vi "运维调试_采配水SNV2.vi"() -> ()   [LabVIEW 2016, in "PLC.lvlib"]
uses:
  PLC.lvlib
  control/switch.ctl
  <vilib>/Plasmionique/MB Master/MB_Master/MB_Master.lvclass
  <vilib>/Utility/miscctls.llb/LVPointTypeDef.ctl
  <vilib>/Plasmionique/MB Master/MB_Master_Serial/MB_Master_Serial.lvclass
  C:/Program Files (x86)/National Instruments/LabVIEW 2016/vi.lib/Plasmionique/MB Master/MB_Master/MB_Master.lvclass
  <vilib>/Plasmionique/MB Master/MB Master.lvlib
panel:
  in  "更新程序 2":T1
  out "X6":bool caption="断电检测"
  out "R13":i16
  in  "进样阀":bool
  in  "更新程序":bool
  in  "R116":i16(ring) caption="储水水体选择" items=["自来水", "采水泵"]
  out "当前启动泵号":u16(ring) items=["1号水样泵", "2号水样泵"]
  out "R113":i16 caption="储水时间设定"
  out "R25":i16
  in  "V14NC":bool
  out "R24":i16
  in  "V14NO":bool
  out "采配水版本号":string
  out "R23":i16 caption="清洗频次计数"
  out "R112":i16 caption="清洗频次设定"
  out "R22":i16
  in  "V13NC":bool
  out "R111":i16 caption="排液时间"
  out "通讯故障":bool
  out "R21":i16
  in  "V13NO":bool
  out "R20":i16
  in  "M1-2":bool
  in  "潜水泵工作模式":u16(ring) items=["泵1单泵单管路", "泵2单泵单管路", "潜水泵双泵双管路", "自吸泵双泵双管路"]
  out "X1":bool caption="进样检测"
  out "X0":bool caption="采样池液位开关"
  out "R109":i16 caption="配水时间"
  out "集成报警信息":string
  out "R108":i16 caption="自来水报警"
  out "R107":i16 caption="采水池液位报警设置"
  out "R106":i16 caption="进样超时设置"
  out "R105":i16 caption="二级清洗时间"
  out "R104":i16 caption="一级清洗时间"
  out "R103":i16 caption="外部管路清洗时间"
  out "R102":i16 caption="静置沉淀时间"
  out "R101":i16 caption="内部管路润洗时间"
  out "R100":i16 caption="外部管路润洗时间"
  out "R2":i16
  out "R1":i16
  out "多列列表框":i32(listbox)
  out "R19":i16
  in  "V6":bool
  out "R18":i16
  in  "V5":bool
  out "R17":i16
  in  "V4":bool
  out "R16":i16
  in  "V3":bool
  out "R15":i16
  in  "V2":bool
  out "R14":i16
  in  "M2":bool
  out "R12":i16
  in  "M1-1":bool
  in  "返回":bool
  in  "参数设置":bool
  in  "单步启动":bool
  in  "启动":bool
  in  "停止":bool
  # "S"
  # "次"
  # "次"
  # "S"
  # "S"
  # "S"
  # "S"
  # "S"
  # "S"
  # "S"
  # "S"
  # "S"
  # "S"
  # "S"
  # "单步计时："
  # "s"
  # "流程计时："
  # "s"
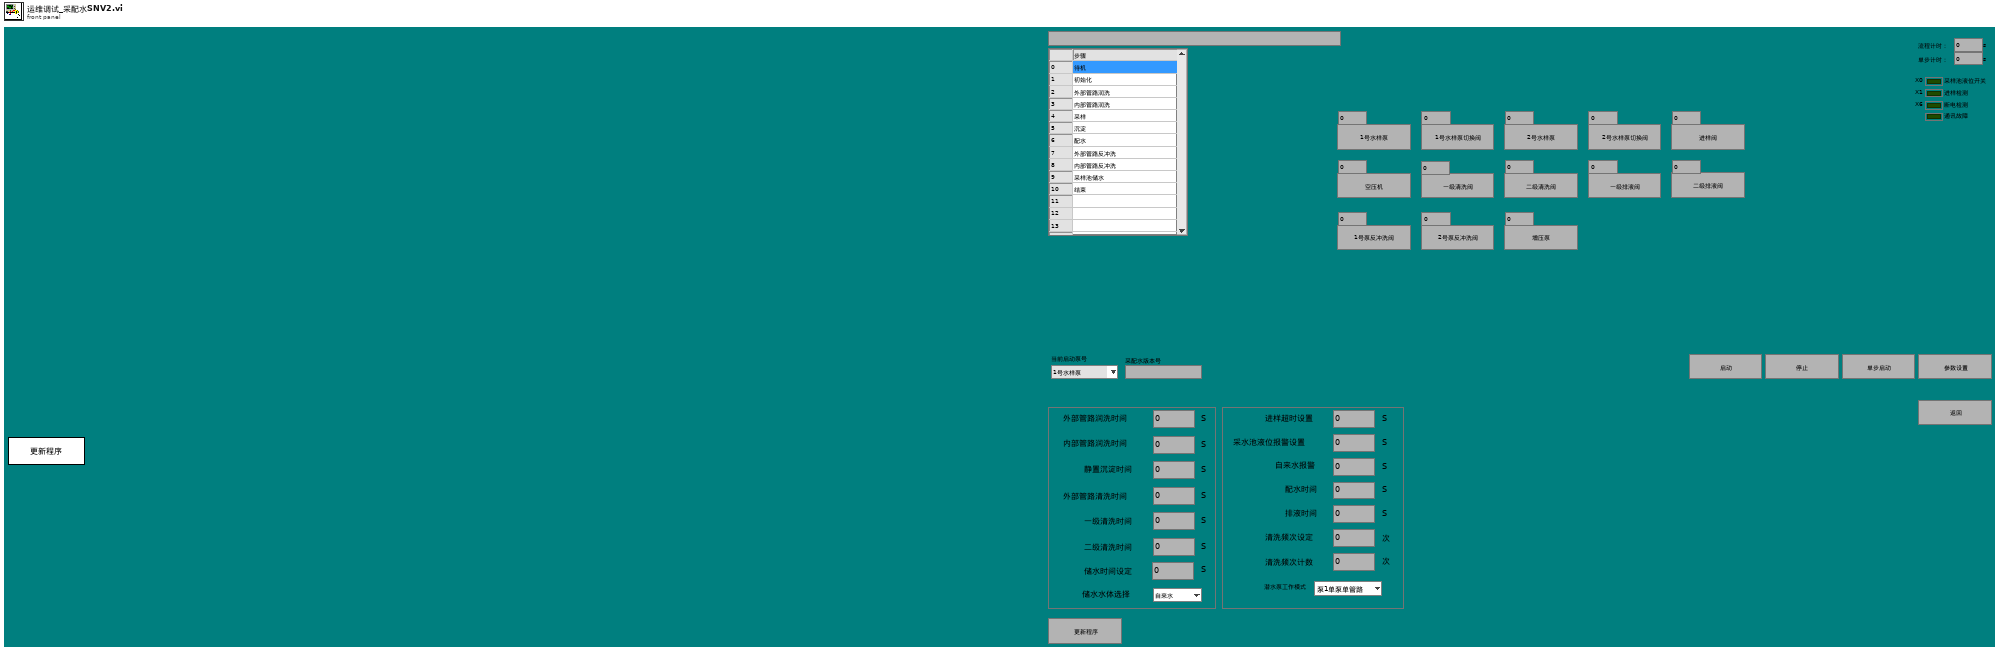
[diagram p1: front panel]
types:
  T1 = typedef "PLC.lvlib/switch.ctl" = bool
  T2 = typedef "参数.ctl" = cluster{"测试模式":enum16{"水样测试", "平行样测试", "集成干预测试", "加标回收"}, "参数启用":T3}
  T3 = typedef "启动参数.ctl" = cluster{"氨氮":bool, "总磷":bool, "总氮":bool, "多参数":bool, "CODmn":bool, "CODCr":bool, "氟化物":bool, "超标留样启用":bool}
  T4 = typedef "LVPointTypeDef.ctl" = cluster{"Horizontal":i16, "Vertical":i16}
  T5 = cluster{"R0":i16, "R1":i16, "R2":i16, "R3":i16, "R4":i16, "R5":i16, "R6":i16, "R7":i16, "R8":i16, "R9":i16, "R10":i16, "R11":i16, "R12":i16, "R13":i16, "R14":i16, "R15":i16, "R16":i16, "R17":i16, "R18":i16, "R19":i16, "R20":i16, "R21":i16, "R22":i16, "R23":i16, "R24":i16, "R25":i16, "R26":i16, "R27":i16, "R28":i16, "R29":i16, "R30":i16, "R31":i16, "R32":i16, "R33":i16, "R34":i16, "R35":i16, "R36":i16, "R37":i16, "R38":i16, "R39":i16, "R40":i16, "R41":i16, "R42":i16, "R43":i16, "R44":i16, "R45":i16, "R46":i16, "R47":i16, "R48":i16, "R49":i16, "R50":i16, "R51":i16, "R52":i16, "R53":i16, "R54":i16, "R55":i16, "R56":i16, "R57":i16, "R58":i16, "R59":i16, "R60":i16, "R61":i16, "R62":i16, "R63":i16, "R64":i16, "R65":i16, "R66":i16, "R67":i16, "R68":i16, "R69":i16, "R70":i16, "R71":i16, "R72":i16, "R73":i16, "R74":i16, "R75":i16, "R76":i16, "R77":i16, "R78":i16, "R79":i16}
  T6 = cluster{"seconds since 1Jan1904":timestamp, "table输入":string, string, "table输入":string}
  T7 = cluster{"命令":string, cluster{"starting address":u16, "holding register value":u16}}
  T8 = cluster{"命令":string, "数据":cluster{"starting address":u16, "holding register value":u16}}
  T9 = cluster{"命令":string, "数据":cluster{"starting address":u16, "holding register values":u16[]}}
  T10 = cluster{"命令":string, "data":cluster{"starting address":u16, "coil values":bool[]}}
  T11 = cluster{"测试模式":enum16{"水样测试", "平行样测试", "集成干预测试", "加标回收"}, "参数启用":T3}
  T12 = cluster{"baud rate (bps)":u32, "stop bits":u16, "parity":u16, "flow control":u16, "timeout":u32, "retries":i32}
  T13 = cluster{"starting address":u16, "holding register values":u16[]}
  T14 = cluster{"starting address":u16, "holding register value":u16}
  T15 = cluster{"starting address":u16, "coil values":bool[]}
  T16 = cluster{"Registers[0]":u16, "Registers[1]":u16, "Registers[2]":u16, "Registers[3]":u16, "Registers[4]":u16, "Registers[5]":u16, "Registers[6]":u16, "Registers[7]":u16, "Registers[8]":u16, "Registers[9]":u16, "Registers[10]":u16, "Registers[11]":u16, "Registers[12]":u16, "Registers[13]":u16, "Registers[14]":u16, "Registers[15]":u16, "Registers[16]":u16, "Registers[17]":u16, "Registers[18]":u16, "Registers[19]":u16, "Registers[20]":u16, "Registers[21]":u16, "Registers[22]":u16, "Registers[23]":u16, "Registers[24]":u16, "Registers[25]":u16, "Registers[26]":u16, "Registers[27]":u16, "Registers[28]":u16, "Registers[29]":u16, "Registers[30]":u16, "Registers[31]":u16, "Registers[32]":u16, "Registers[33]":u16, "Registers[34]":u16, "Registers[35]":u16, "Registers[36]":u16, "Registers[37]":u16, "Registers[38]":u16, "Registers[39]":u16, "Registers[40]":u16, "Registers[41]":u16, "Registers[42]":u16, "Registers[43]":u16, "Registers[44]":u16, "Registers[45]":u16, "Registers[46]":u16, "Registers[47]":u16, "Registers[48]":u16, "Registers[49]":u16, "Registers[50]":u16, "Registers[51]":u16, "Registers[52]":u16, "Registers[53]":u16, "Registers[54]":u16, "Registers[55]":u16, "Registers[56]":u16, "Registers[57]":u16, "Registers[58]":u16, "Registers[59]":u16, "Registers[60]":u16, "Registers[61]":u16, "Registers[62]":u16, "Registers[63]":u16, "Registers[64]":u16, "Registers[65]":u16, "Registers[66]":u16, "Registers[67]":u16, "Registers[68]":u16, "Registers[69]":u16, "Registers[70]":u16, "Registers[71]":u16, "Registers[72]":u16, "Registers[73]":u16, "Registers[74]":u16, "Registers[75]":u16, "Registers[76]":u16, "Registers[77]":u16, "Registers[78]":u16, "Registers[79]":u16}
  T17 = cluster{"Registers[0]":u16, "Registers[1]":u16, "Registers[2]":u16, "Registers[3]":u16, "Registers[4]":u16, "Registers[5]":u16}
  T18 = cluster{"Registers[0]":u16, "Registers[1]":u16, "Registers[2]":u16, "Registers[3]":u16, "Registers[4]":u16, "Registers[5]":u16, "Registers[6]":u16, "Registers[7]":u16, "Registers[8]":u16, "Registers[9]":u16, "Registers[10]":u16, "Registers[11]":u16, "Registers[12]":u16, "Registers[13]":u16, "Registers[14]":u16, "Registers[15]":u16, "Registers[16]":u16, "Registers[17]":u16, "Registers[18]":u16, "Registers[19]":u16, "Registers[20]":u16, "Registers[21]":u16, "Registers[22]":u16, "Registers[23]":u16, "Registers[24]":u16, "Registers[25]":u16, "Registers[26]":u16, "Registers[27]":u16, "Registers[28]":u16, "Registers[29]":u16, "Registers[30]":u16, "Registers[31]":u16, "Registers[32]":u16, "Registers[33]":u16}
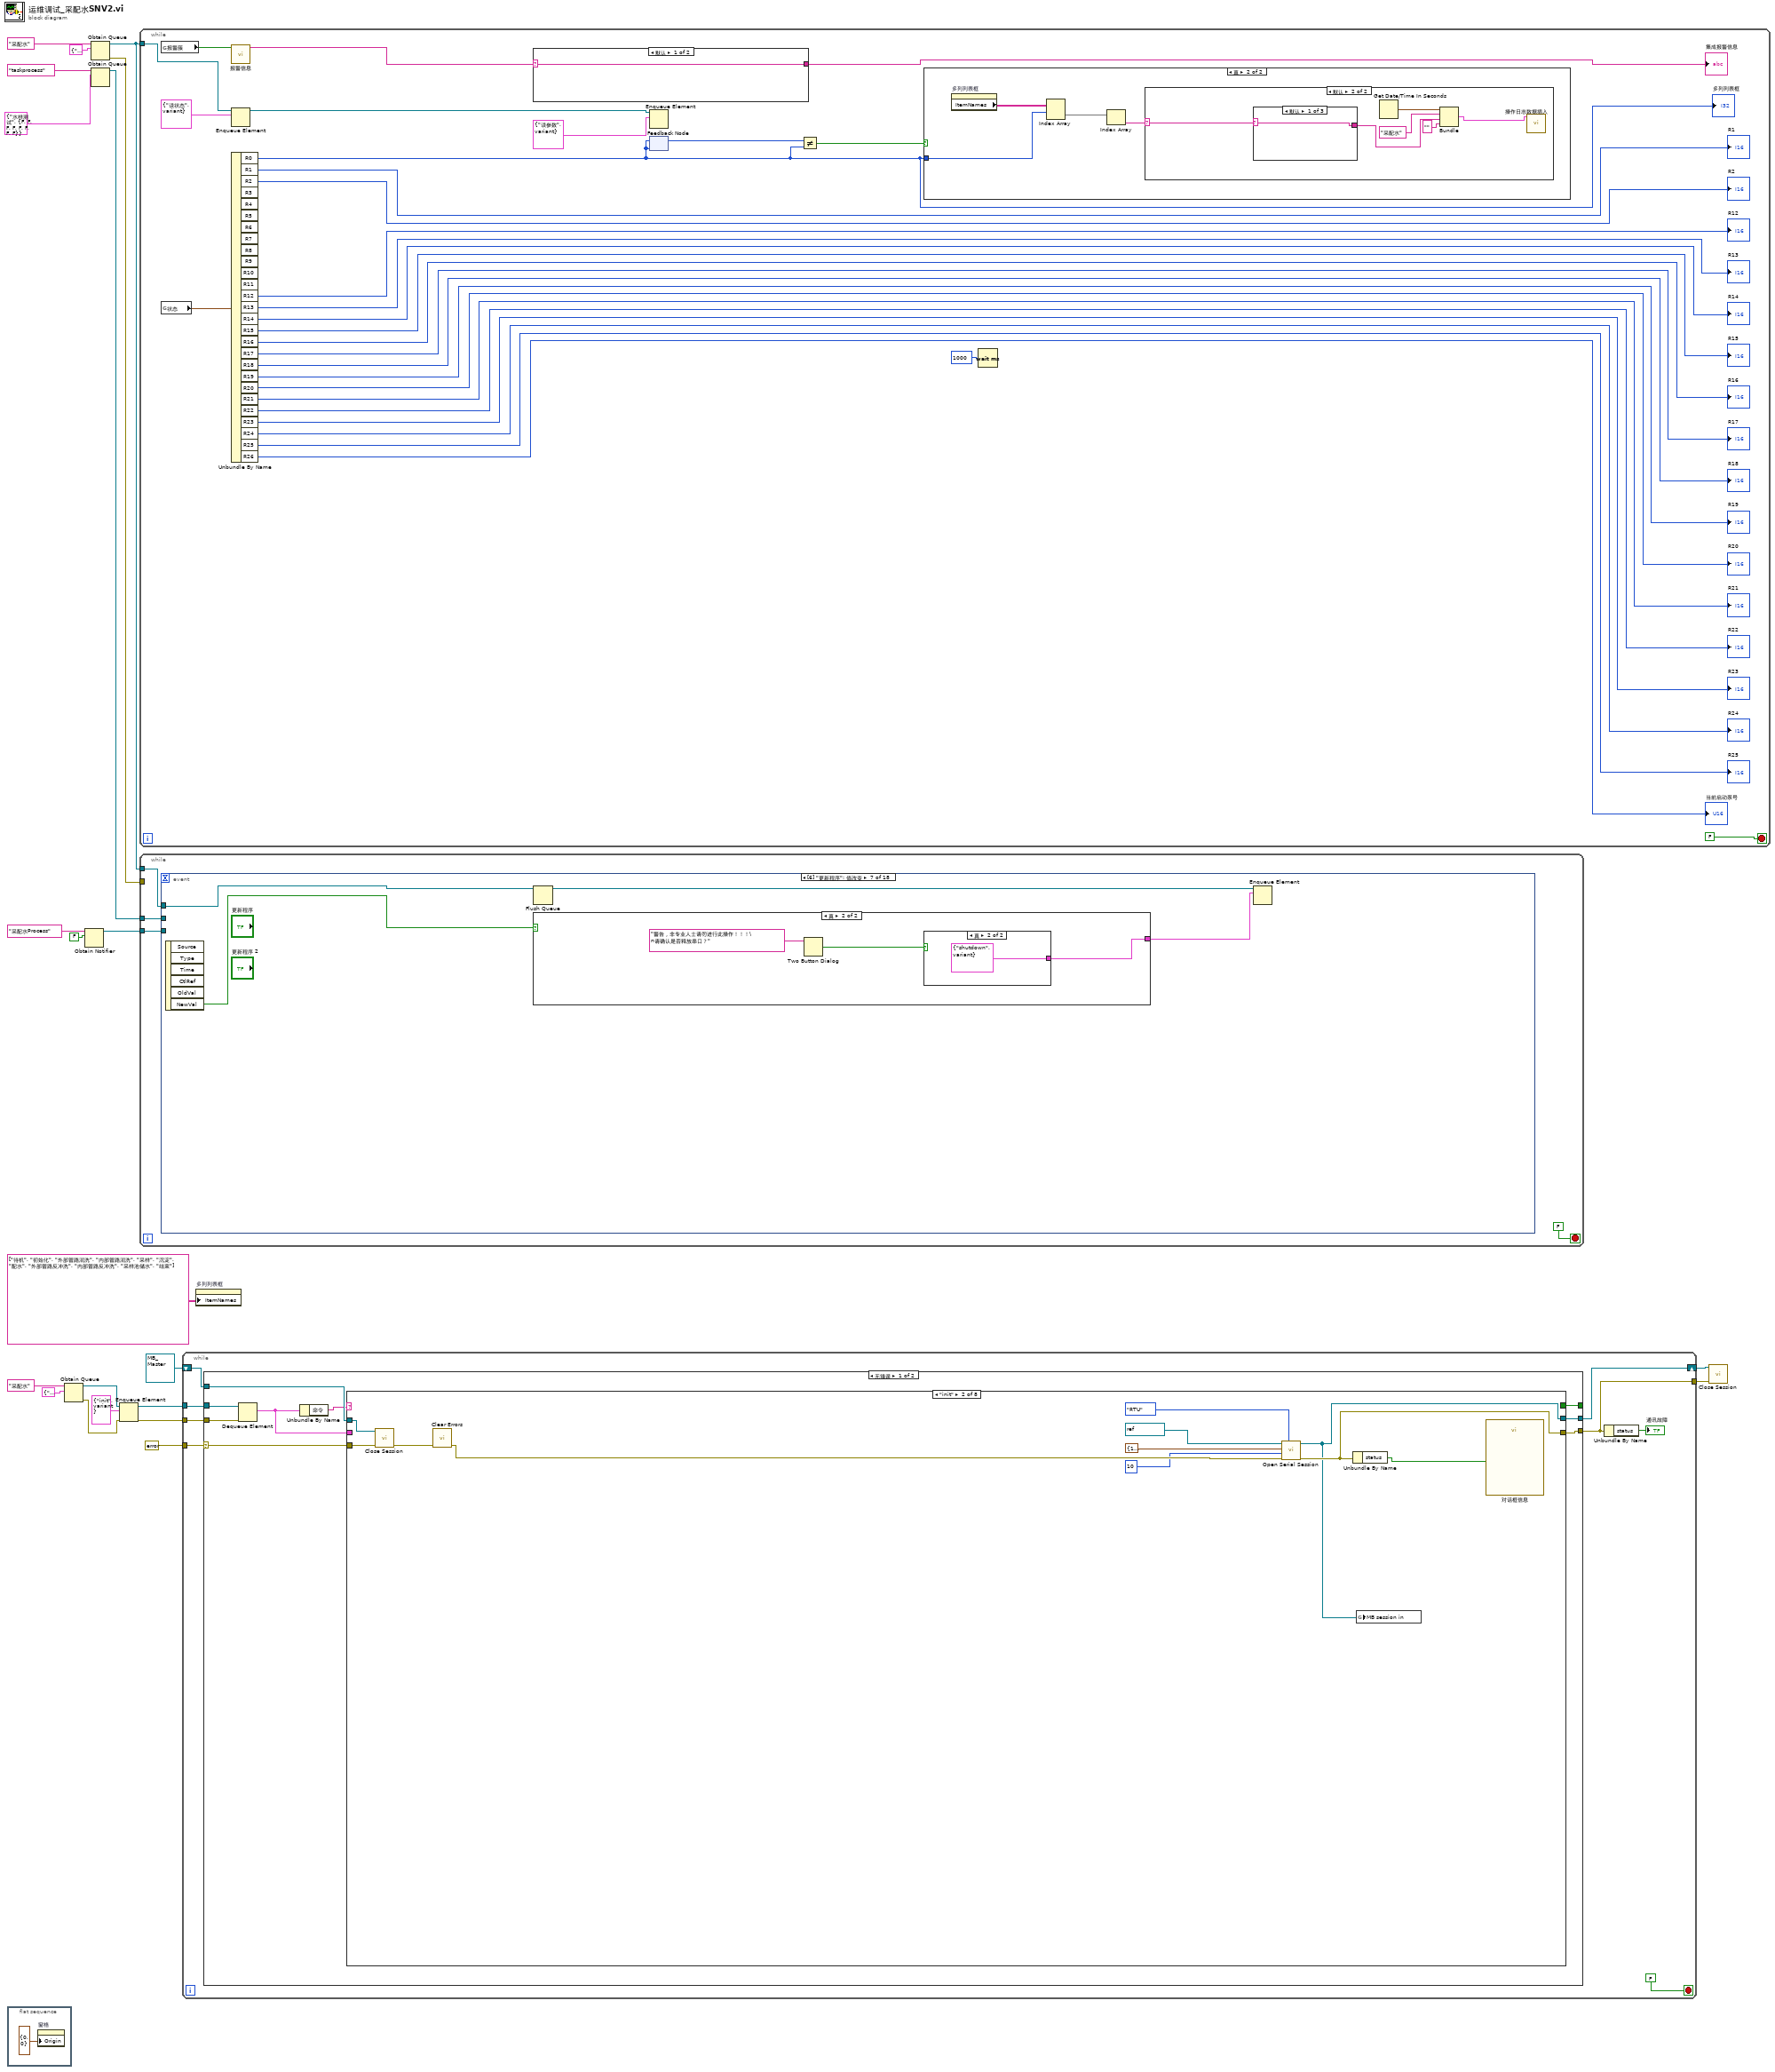
[diagram p0: block diagram]
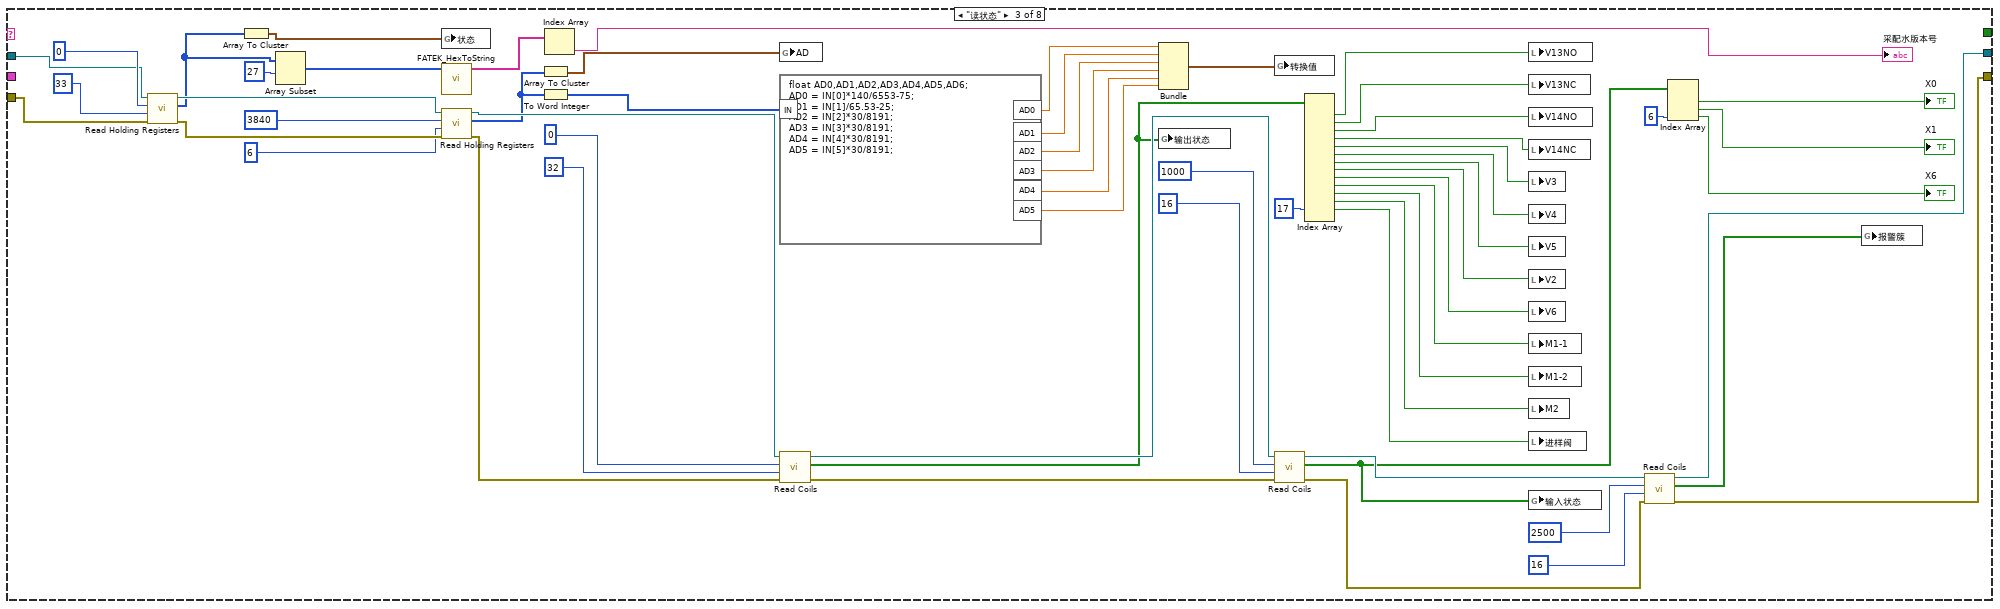
[diagram p3: hidden frame]
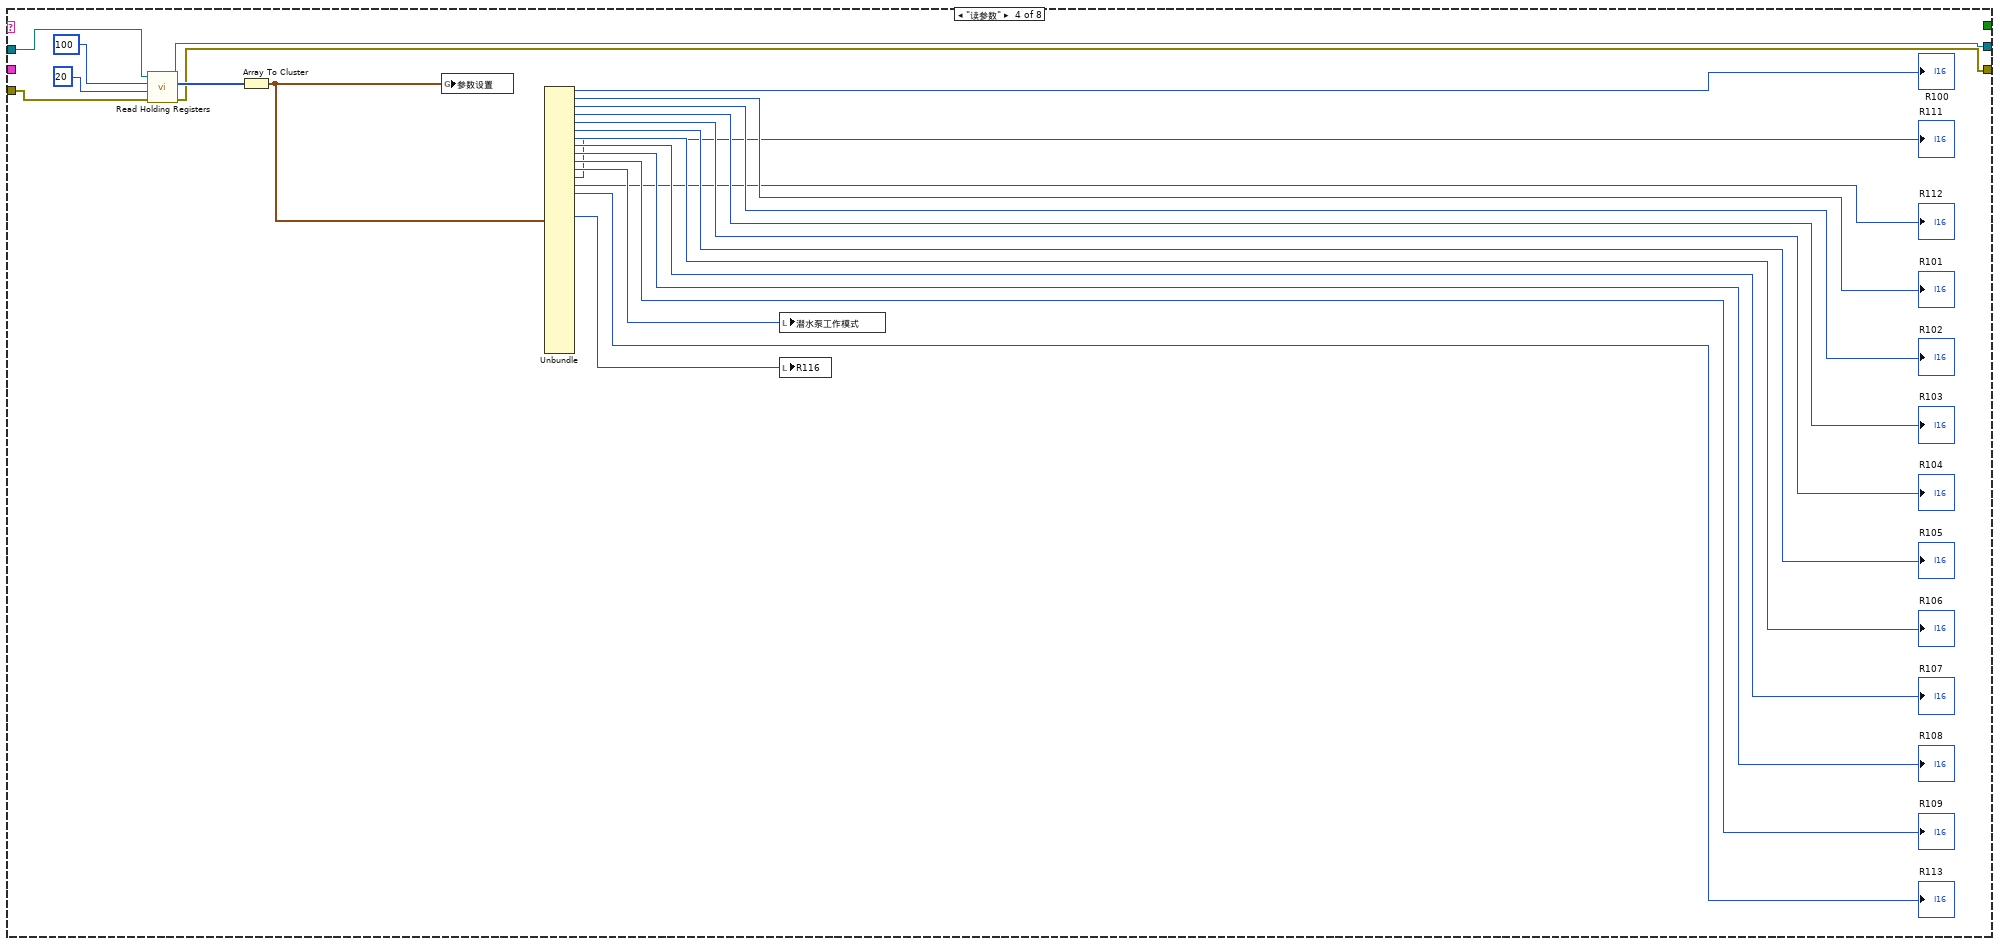
[diagram p4: hidden frame]
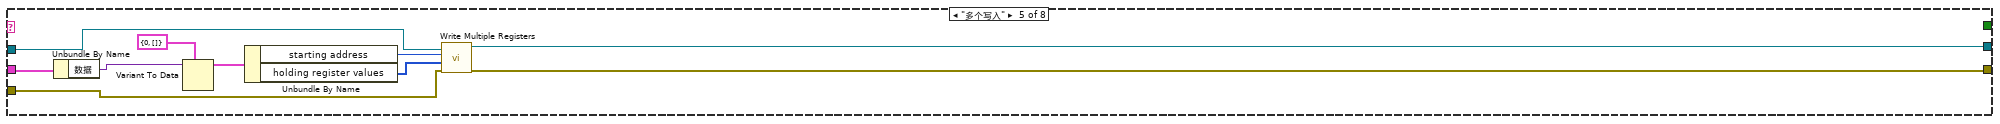
[diagram p5: hidden frame]
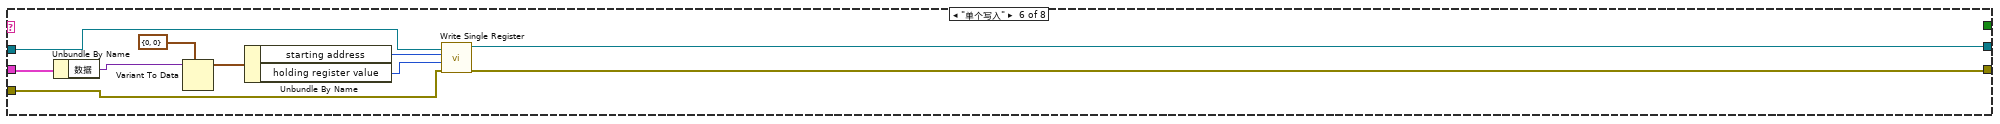
[diagram p6: hidden frame]
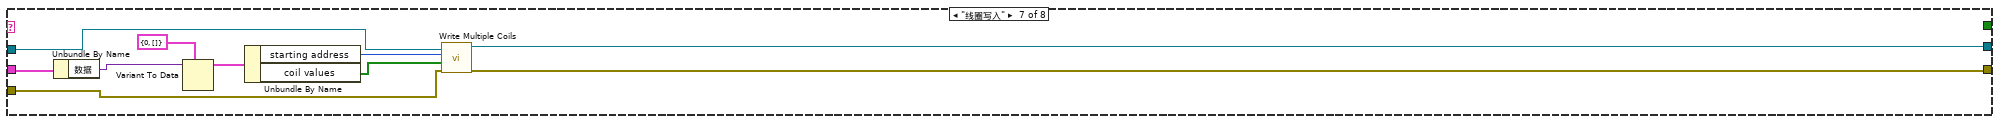
[diagram p7: hidden frame]
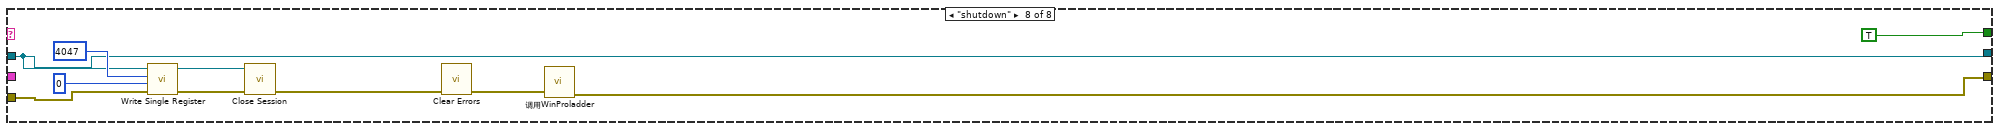
[diagram p8: hidden frame]
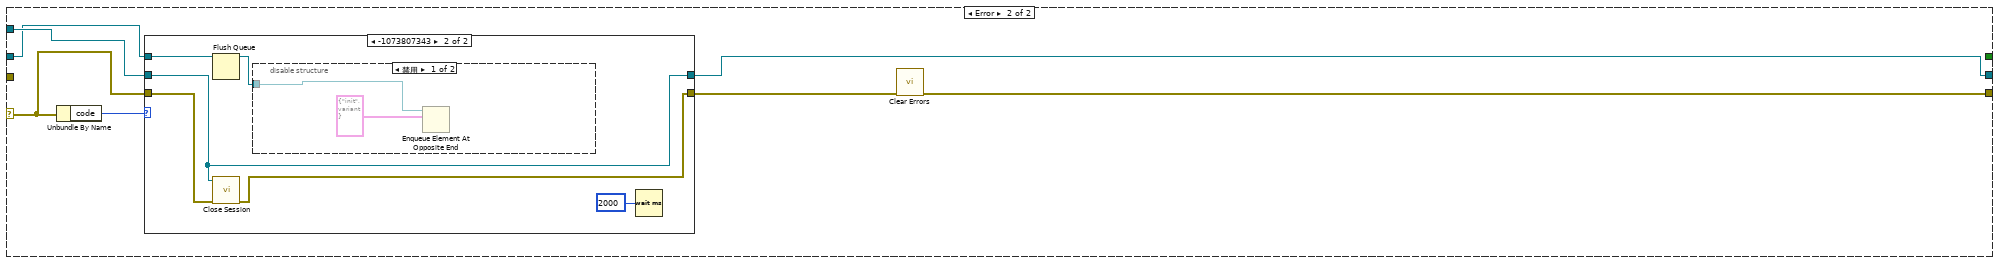
[diagram p9: hidden frame]
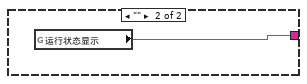
[diagram p12: hidden frame]
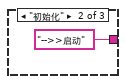
[diagram p15: hidden frame]
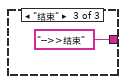
[diagram p16: hidden frame]
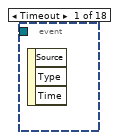
[diagram p17: hidden frame]
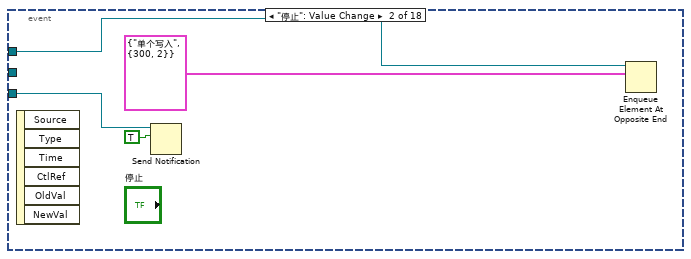
[diagram p18: hidden frame]
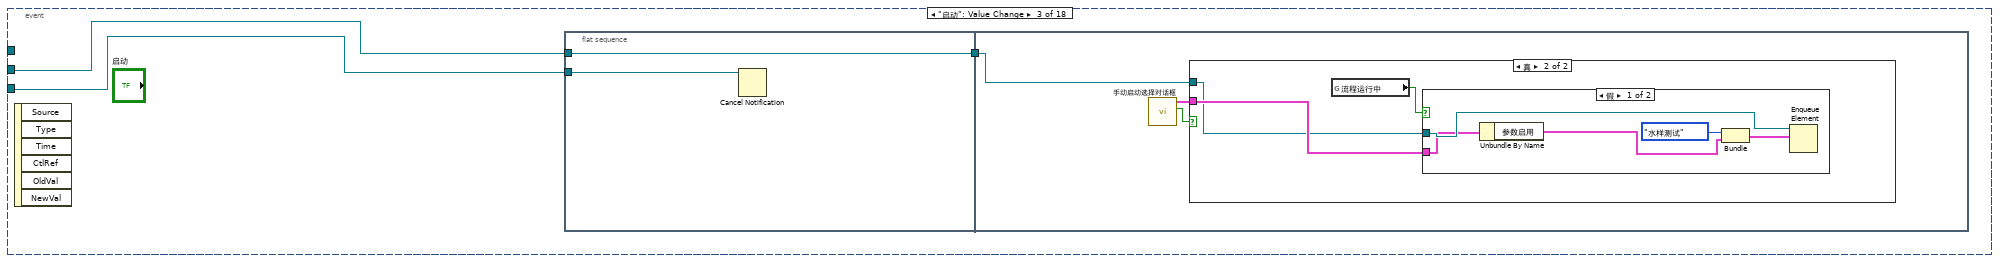
[diagram p19: hidden frame]
diagram:
  n1 = flat-sequence {
    frame #0 {
      n2 = property on="窗格" class="Pane"("Origin"=T4 {"Horizontal"=0, "Vertical"=0} ("原点")) -> ()  [unwired: 2 in, 2 out]
    }
  }
  n3 = Obtain Queue(name (unnamed)="采配水" ("名称（未命名）"), element data type=cluster{"命令":string, "数据":variant} {"命令"="", "数据"=variant}) -> (queue out=w12:refnum<queue>, error out=w11:errorcluster)  [unwired: 3 in, 1 out]
  n4 = Obtain Notifier(name (unnamed)="采配水Process" ("名称（未命名）"), notification data type=FALSE) -> (notifier out=w15:refnum<notifier>)  [unwired: 2 in, 2 out]
  n5 = Obtain Queue(name (unnamed)="采配水" ("名称（未命名）"), element data type=cluster{"命令":string, "数据":variant} {"命令"="", "数据"=variant}) -> (queue out=w19:refnum<queue>, error out=w20:errorcluster)  [unwired: 3 in, 1 out]
  n6 = Obtain Queue(name (unnamed)="taskprocess" ("名称（未命名）"), element data type=T2 {"测试模式"=enum."水样测试", "参数启用"={"氨氮"=FALSE, "总磷"=FALSE, "总氮"=FALSE, "多参数"=FALSE, "CODmn"=FALSE, "CODCr"=FALSE, "氟化物"=FALSE, "超标留样启用"=FALSE}} ("参数")) -> (queue out=w2:refnum<queue>)  [unwired: 3 in, 2 out]
  n7 = Enqueue Element(queue=w12, element=cluster{"命令":string, "数据":variant} {"命令"="init", "数据"=variant} ("元素"), error in (no error)=w11) -> (queue out=w7:refnum<queue>, error out=w9:errorcluster)  [unwired: 1 in, 1 out]
  n8 = while {
    tunnel: w19 -> [w52]
    stop <- FALSE stop-if-true
    n9 = global read "采配水全局变量.vi" "报警簇"() -> (w39:bool[])
    n10 = global read "采配水全局变量.vi" "状态"() -> (w50:T5)
    n11 = call "报警信息.vi"("报警簇"=w39) -> ("采配水报警信息"=w32:string)  [unwired: 9 in, 1 out]
    n12 = Enqueue Element(queue=w52, element=cluster{"命令":string, "数据":variant} {"命令"="读状态", "数据"=variant} ("元素")) -> (queue out=w35:refnum<queue>)  [unwired: 2 in, 2 out]
    n13 = Unbundle By Name(w50) -> ("R0"=w33:i16, "R1"=→"R1":i16, "R2"=→"R2":i16, "R12"=→"R12":i16, "R13"=→"R13":i16, "R14"=→"R14":i16, "R15"=→"R15":i16, "R16"=→"R16":i16, "R17"=→"R17":i16, "R18"=→"R18":i16, "R19"=→"R19":i16, "R20"=→"R20":i16, "R21"=→"R21":i16, "R22"=→"R22":i16, "R23"=→"R23":i16, "R24"=→"R24":i16, "R25"=→"R25":i16, "R26"=→"当前启动泵号":i16)  [unwired: 9 out]
    "多列列表框" <- w33
    n14 = case shown="默认" w32 {
      selector: w32 -> [w54 _]
      tunnel: [w54 w55] -> w38
      frame Default {
      }
      frame "" {
        n15 = global read "采配水全局变量.vi" "运行状态显示"() -> (w55:string)
      }
    }
    "集成报警信息" <- w38
    n16 = Enqueue Element(queue=w35, element=cluster{"命令":string, "数据":variant} {"命令"="读参数", "数据"=variant} ("元素")) -> ()  [unwired: 2 in, 3 out]
    n17 = feedback-in #1(w33) -> ()
    n18 = feedback #1(w33) -> (w34:i16)
    n19 = Not Equal?(x=w34, y=w33) -> (x != y?=w40:bool)
    n20 = case shown="真" w40 {
      tunnel: w33 -> [_ w58]
      frame False {
      }
      frame True {
        n21 = property on="多列列表框" class="MCListbox (严格)"() -> ("ItemNames"=w59:string[][])  [unwired: 2 in, 2 out]
        n22 = Index Array(array=w59, index (row)=w58) -> (element=w57:string[])  [unwired: 1 in]
        n23 = Index Array(array=w57) -> (element=w56:string)  [unwired: 1 in]
        n24 = case shown="默认" w56 {
          selector: w56 -> [_ w62]
          frame "待机" {
          }
          frame Default {
            n25 = case shown="默认" w62 {
              selector: w62 -> [w66 _ _]
              tunnel: [w66 "-->>启动" "-->>结束"] -> w61
              frame Default {
              }
              frame "初始化" {
              }
              frame "结束" {
              }
            }
            n26 = Get Date/Time In Seconds() -> (seconds since 1Jan1904=w65:timestamp)
            n27 = Bundle("seconds since 1Jan1904"=w65, "table输入"="采配水", w61, "table输入"="") -> (w60:T6)  [unwired: 1 in]
            n28 = call "操作日志数据插入.vi"("data"=w60) -> ()  [unwired: 9 in, 1 out]
          }
        }
      }
    }
    n29 = Wait (ms)(milliseconds to wait=u32 1000 ("等待时间（毫秒）")) -> ()  [unwired: 1 out]
  }
  n30 = while {
    tunnel: w19 -> [w71]
    tunnel: w20 -> [_]
    tunnel: w15 -> [w70]
    tunnel: w2 -> [w69]
    stop <- FALSE stop-if-true
    n31 = event shown="[6] \"更新程序\": 值改变" {
      selector: _ -> [_ _ _ _ _ _ _ _ _ _ _ _ _ _ _ _ _ _]
      dyn-events: _ -> [_ _ _ _ _ _ _ _ _ _ _ _ _ _ _ _ _ _]
      timeout: _ -> [_ _ _ _ _ _ _ _ _ _ _ _ _ _ _ _ _ _]
      tunnel: w71 -> [_ w75 _ w97 w116 w119 w124 w135 _ _ _ _ w163 w165 w170 w175 w180 w185]
      tunnel: w70 -> [_ w74 w79 _ _ _ _ _ _ _ _ _ _ _ _ _ _ _]
      tunnel: w69 -> [_ _ w77 _ _ _ _ _ _ _ _ _ _ _ _ _ _ _]
      event Timeout {
        n32 = event-data() -> ()  [unwired: 1 in, 3 out]
      }
      event "停止": Value Change {
        n33 = event-data() -> ()  [unwired: 1 in, 6 out]
        n34 = Send Notification(notification=TRUE ("通知"), notifier=w74) -> ()  [unwired: 1 in, 2 out]
        n35 = Enqueue Element At Opposite End(queue=w75, element=T7 {"命令"="单个写入", {"starting address"=300, "holding register value"=2}} ("元素")) -> ()  [unwired: 2 in, 3 out]
      }
      event "启动": Value Change {
        n36 = event-data() -> ()  [unwired: 1 in, 6 out]
        n37 = flat-sequence {
          tunnel: w79 -> [w81]
          tunnel: [w80] -> w78
          tunnel: w77 -> [w80]
          tunnel: w78 -> [w82]
          frame #0 {
            n38 = Cancel Notification(0:w81) -> ()  [unwired: 1 in, 3 out]
          }
          frame #1 {
            n39 = call "手动启动选择对话框.vi"() -> ("确定"=w84:bool, "输出簇"=w83:cluster{"参数启用":T3})  [unwired: 10 in]
            n40 = case shown="真" w84 {
              tunnel: w83 -> [_ w86]
              tunnel: w82 -> [_ w85]
              frame False {
              }
              frame True {
                n41 = global read "采配水全局变量.vi" "流程运行中"() -> (w87:bool)
                n42 = case shown="假" w87 {
                  tunnel: w86 -> [w90 _]
                  tunnel: w85 -> [w92 _]
                  frame False {
                    n43 = Unbundle By Name(w90) -> ("参数启用"=w89:T3)
                    n44 = Bundle("测试模式"=enum16{"水样测试", "平行样测试", "集成干预测试", "加标回收"}."水样测试", "参数启用"=w89) -> (w88:T11)  [unwired: 1 in]
                    n45 = Enqueue Element(queue=w92, element=w88) -> ()  [unwired: 2 in, 3 out]
                  }
                  frame True {
                    n46 = One Button Dialog(message="流程已启动，无需重复启动！" ("消息")) -> ()  [unwired: 1 in, 1 out]
                  }
                }
              }
            }
          }
        }
      }
      event "单步启动": Value Change {
        n47 = event-data() -> ()  [unwired: 1 in, 6 out]
        n48 = call "单步启动对话框.vi"() -> ("单步启动步骤输出"=w94:u16)  [unwired: 11 in]
        n49 = Bundle By Name(cluster=T8 {"命令"="单个写入", "数据"={"starting address"=301, "holding register value"=0}} ("元素"), "数据.holding register value"=w94) -> (w95:T8)
        n50 = Enqueue Element At Opposite End(queue=w97, element=w95) -> ()  [unwired: 2 in, 3 out]
      }
      event "R100", "R101", "R102", "R103", "R104", "R105", "R106", "R107", "R108", "R109", "潜水泵工作模式", "R111", "R112", "R113": Value Change {
        n51 = event-data() -> ()  [unwired: 1 in, 6 out]
        n52 = local read "R100"() -> (w111:i16)
        n53 = local read "R101"() -> (w110:i16)
        n54 = local read "R102"() -> (w109:i16)
        n55 = local read "R103"() -> (w108:i16)
        n56 = local read "R104"() -> (w107:i16)
        n57 = local read "R105"() -> (w106:i16)
        n58 = local read "R106"() -> (w105:i16)
        n59 = local read "R107"() -> (w104:i16)
        n60 = local read "R108"() -> (w103:i16)
        n61 = local read "R109"() -> (w102:i16)
        n62 = local read "R111"() -> (w100:i16)
        n63 = local read "R112"() -> (w99:i16)
        n64 = local read "R113"() -> (w98:i16)
        n65 = Build Array(w111, w110, w109, w108, w107, w106, w105, w104, w103, w102, "潜水泵工作模式", w100, w99, w98) -> (w112:u16[])
        n66 = Bundle By Name(cluster=T9 {"命令"="多个写入", "数据"={"starting address"=0, "holding register values"=[]}} ("元素"), "数据.starting address"=u16 100, "数据.holding register values"=w112) -> (w113:T9)
        n67 = Enqueue Element At Opposite End(queue=w116, element=w113) -> ()  [unwired: 2 in, 3 out]
      }
      event "R116": Value Change {
        n68 = event-data() -> ()  [unwired: 1 in, 6 out]
        n69 = Build Array("R116") -> (w118:i16[])
        n70 = Bundle By Name(cluster=T9 {"命令"="多个写入", "数据"={"starting address"=0, "holding register values"=[]}} ("元素"), "数据.starting address"=u16 116, "数据.holding register values"=w118) -> (w120:T9)
        n71 = Enqueue Element At Opposite End(queue=w119, element=w120) -> ()  [unwired: 2 in, 3 out]
      }
      event "更新程序": Value Change {
        n72 = event-data() -> ("NewVal"=w123:bool)  [unwired: 1 in, 5 out]
        n73 = Flush Queue(queue=w124) -> (queue out=w125:refnum<queue>)  [unwired: 1 in, 2 out]
        n74 = case shown="真" w123 {
          tunnel: [cluster{"命令":string, "数据":variant} {"命令"="init", "数据"=variant} ("元素") w130] -> w126
          frame False {
          }
          frame True {
            n75 = Two Button Dialog(message="警告，非专业人士请勿进行此操作！！！\n请确认是否释放串口？" ("消息")) -> (T button?=w129:bool)  [unwired: 2 in]
            n76 = case shown="真" w129 {
              tunnel: [_ cluster{"命令":string, "数据":variant} {"命令"="shutdown", "数据"=variant} ("元素")] -> w130
              frame False {
                n77 = local write "更新程序 2"(FALSE ("释放串口")) -> ()
              }
              frame True {
              }
            }
          }
        }
        n78 = Enqueue Element(queue=w125, element=w126) -> ()  [unwired: 2 in, 3 out]
      }
      event "R23": Value Change {
        n79 = event-data() -> ()  [unwired: 1 in, 6 out]
        n80 = local read "R23"() -> (w134:i16)
        n81 = Build Array(w134) -> (w133:i16[])
        n82 = Bundle By Name(cluster=T9 {"命令"="多个写入", "数据"={"starting address"=0, "holding register values"=[]}} ("元素"), "数据.starting address"=u16 23, "数据.holding register values"=w133) -> (w136:T9)
        n83 = Enqueue Element At Opposite End(queue=w135, element=w136) -> ()  [unwired: 2 in, 3 out]
      }
      event "R23": Mouse Down {
        n84 = event-data() -> ("CtlRef"=w141:refnum<vi>)  [unwired: 1 in, 7 out]
        n85 = Two Button Dialog(message="请确认是否更改，更改后将影响实际清洗频次" ("消息")) -> (T button?=w140:bool)  [unwired: 2 in]
        n86 = case shown="真" w140 {
          tunnel: w141 -> [_ w142]
          frame False {
          }
          frame True {
            n87 = property class="DigNum (严格)"(reference=w142) -> (reference out=w144:refnum<vi>, "Value"=w145:i16)  [unwired: 1 in, 1 out]
            n88 = call "数字键盘.vi"("OldNumber"=w145) -> ("NewNumber"=w143:sgl)
            n89 = property class="DigNum (严格)"(reference=w144, "Val(Sgnl)"=w143) -> ()  [unwired: 1 in, 2 out]
          }
        }
      }
      event "R100", "R101", "R102", "R103", "R104", "R105", "R106", "R107", "R108", "R109", "R111", "R112", "R113": Mouse Down {
        n90 = event-data() -> ("CtlRef"=w149:refnum<vi>)  [unwired: 1 in, 7 out]
        n91 = property class="DigNum (严格)"(reference=w149) -> (reference out=w147:refnum<vi>, "Value"=w148:i16)  [unwired: 1 in, 1 out]
        n92 = call "数字键盘.vi"("OldNumber"=w148) -> ("NewNumber"=w146:sgl)
        n93 = property class="DigNum (严格)"(reference=w147, "Val(Sgnl)"=w146) -> ()  [unwired: 1 in, 2 out]
      }
      event "参数设置": Value Change {
        n94 = event-data() -> ()  [unwired: 1 in, 6 out]
        n95 = property on="窗格" class="Pane"("Origin"=T4 {"Horizontal"=0, "Vertical"=628} ("原点")) -> ()  [unwired: 2 in, 2 out]
      }
      event "返回": Value Change {
        n96 = event-data() -> ()  [unwired: 1 in, 6 out]
        n97 = property on="窗格" class="Pane"("Origin"=T4 {"Horizontal"=0, "Vertical"=0} ("原点")) -> ()  [unwired: 2 in, 2 out]
      }
      event "M1-1", "M2", "V2", "V3", "V4", "V5", "V6", "进样阀": Value Change {
        n98 = event-data() -> ()  [unwired: 1 in, 6 out]
        n99 = Build Array("M1-1", "进样阀", "M2", "V2", "V3", "V4", "V5", "V6") -> (w155:bool[])
        n100 = Bundle By Name(cluster=T10 {"命令"="线圈写入", "data"={"starting address"=2400, "coil values"=[]}} ("元素"), "data.coil values"=w155) -> (w156:T10)
        n101 = Enqueue Element(queue=w163, element=w156) -> ()  [unwired: 2 in, 3 out]
      }
      event "M1-2": Value Change {
        n102 = event-data() -> ()  [unwired: 1 in, 6 out]
        n103 = Build Array("M1-2") -> (w166:bool[])
        n104 = Bundle By Name(cluster=T10 {"命令"="线圈写入", "data"={"starting address"=2413, "coil values"=[]}} ("元素"), "data.coil values"=w166) -> (w167:T10)
        n105 = Enqueue Element(queue=w165, element=w167) -> ()  [unwired: 2 in, 3 out]
      }
      event "V13NO": Value Change {
        n106 = event-data() -> ()  [unwired: 1 in, 6 out]
        n107 = Build Array("V13NO") -> (w171:bool[])
        n108 = Bundle By Name(cluster=T10 {"命令"="线圈写入", "data"={"starting address"=2414, "coil values"=[]}} ("元素"), "data.coil values"=w171) -> (w172:T10)
        n109 = Enqueue Element(queue=w170, element=w172) -> ()  [unwired: 2 in, 3 out]
      }
      event "V13NC": Value Change {
        n110 = event-data() -> ()  [unwired: 1 in, 6 out]
        n111 = Build Array("V13NC") -> (w176:bool[])
        n112 = Bundle By Name(cluster=T10 {"命令"="线圈写入", "data"={"starting address"=2415, "coil values"=[]}} ("元素"), "data.coil values"=w176) -> (w177:T10)
        n113 = Enqueue Element(queue=w175, element=w177) -> ()  [unwired: 2 in, 3 out]
      }
      event "V14NO": Value Change {
        n114 = event-data() -> ()  [unwired: 1 in, 6 out]
        n115 = Build Array("V14NO") -> (w181:bool[])
        n116 = Bundle By Name(cluster=T10 {"命令"="线圈写入", "data"={"starting address"=2408, "coil values"=[]}} ("元素"), "data.coil values"=w181) -> (w182:T10)
        n117 = Enqueue Element(queue=w180, element=w182) -> ()  [unwired: 2 in, 3 out]
      }
      event "V14NC": Value Change {
        n118 = event-data() -> ()  [unwired: 1 in, 6 out]
        n119 = Build Array("V14NC") -> (w186:bool[])
        n120 = Bundle By Name(cluster=T10 {"命令"="线圈写入", "data"={"starting address"=2409, "coil values"=[]}} ("元素"), "data.coil values"=w186) -> (w187:T10)
        n121 = Enqueue Element(queue=w185, element=w187) -> ()  [unwired: 2 in, 3 out]
      }
    }
  }
  n122 = while {
    tunnel: w7 -> [w193]
    tunnel: w9 -> [w192]
    shift-right: [w196] -> w4
    shift-left: refnum<class "MB_Master.lvclass"> refnum ("MB session in") -> [w195]
    tunnel: errorcluster {"status"=FALSE, "code"=0, "source"=""} ("error out") -> [w194]
    tunnel: [w191] -> w5
    stop <- FALSE stop-if-true
    n123 = case shown="无错误" w194 {
      selector: w194 -> [w202 w345]
      tunnel: [w205 w344] -> w196
      tunnel: w195 -> [w204 w346]
      tunnel: [w203 w342] -> w191
      tunnel: w193 -> [w199 w341]
      tunnel: w192 -> [w198 _]
      tunnel: [w200 _] -> _
      frame No Error {
        n124 = Dequeue Element(queue=w199, error in (no error)=w198) -> (element=w197:cluster{"命令":string, "数据":variant})  [unwired: 1 in, 3 out]
        n125 = Unbundle By Name(w197) -> ("命令"=w201:string)
        n126 = case shown="\"init\"" w201 {
          tunnel: [w207 w208 w247 w295 w307 w317 w327 w333] -> w205
          tunnel: w204 -> [w207 w215 w265 w300 w310 w320 w330 w333]
          tunnel: [w206 w213 w246 w294 w308 w318 w328 w331] -> w203
          tunnel: w202 -> [w206 w217 w268 w299 w309 w319 w329 w334]
          tunnel: [_ _ _ _ _ _ _ TRUE] -> w200
          tunnel: w197 -> [_ _ _ _ w306 w316 w326 _]
          frame "idle", Default {
          }
          frame "init" {
            n127 = call-dynamic "Close Session.vi"("error in (no error)"=w217, "MB session in"=w215) -> ("error out"=w216:errorcluster)  [unwired: 9 in]
            n128 = call <vilib>:"Clear Errors.vi"("error in (no error)"=w216) -> ("error out"=w214:errorcluster)  [unwired: 5 in, 1 out]
            n129 = call <vilib>:"Open Serial Session.vi"("Mode (RTU)"=enum16{"RTU", "ASCII"}."RTU", "Error in"=w214, "Slave ID"=u8 10, "Serial Config"=T12 {"baud rate (bps)"=115200, "stop bits"=10, "parity"=0, "flow control"=0, "timeout"=500, "retries"=1}, "VISA Resource"=refnum<visa-resource-name> "COM3" ("VISA resource name")) -> ("Error out"=w213:errorcluster, "MB_Serial session"=w208:refnum<class "MB_Master_Serial.lvclass">)  [unwired: 5 in]
            n130 = Unbundle By Name(w213) -> ("status"=w218:bool)
            n131 = global write "采配水全局变量.vi" "MB session in"(w208) -> ()
            n132 = call "对话框信息"("Enable"=w218) -> ()  [unwired: 9 in, 2 out]
          }
          frame "读状态" {
            n133 = call <vilib>:"Read Holding Registers.vi"("error in (no error)"=w268, "quantity"=u16 33 ("number of holding registers"), "starting address"=u16 0, "MB session in"=w265) -> ("error out"=w263:errorcluster, "Registers"=w241:u16[], "MB session out"=w264:refnum<class "MB_Master.lvclass">)  [unwired: 5 in]
            n134 = Array To Cluster(array=w241) -> (cluster=w269:T16)
            n135 = Array Subset(array=w241, index=27 ("索引")) -> (w239:u16[])  [unwired: 1 in]
            n136 = global write "采配水全局变量.vi" "状态"(w269) -> ()
            n137 = call "FATEK_HexToString.vi"("数组"=w239) -> ("STRING"=w238:string[])  [unwired: 10 in]
            n138 = call <vilib>:"Read Holding Registers.vi"("error in (no error)"=w263, "quantity"=u16 6 ("number of holding registers"), "starting address"=u16 3840, "MB session in"=w264) -> ("error out"=w259:errorcluster, "Registers"=w243:u16[], "MB session out"=w260:refnum<class "MB_Master.lvclass">)  [unwired: 5 in]
            n139 = Array To Cluster(array=w243) -> (cluster=w277:T17)
            n140 = To Word Integer(number=w243) -> (16bit integer=w242:i16[])
            n141 = Index Array(array=w238) -> (element=→"采配水版本号":string)  [unwired: 1 in]
            n142 = global write "采配水全局变量.vi" "AD"(w277) -> ()
            n143 = formula code="float AD0,AD1,AD2,AD3,AD4,AD5,AD6;\nAD0 = IN[0]*140/6553-75;\nAD1 = IN[1]/65.53-25;\nAD2 = IN[2]*30/8191;\nAD3 = IN[3]*30/8191;\nAD4 = IN[4]*30/8191;\nAD5 = IN[5]*30/8191;"("IN"=w242) -> ("AD0"=w275:dbl, "AD1"=w274:dbl, "AD2"=w273:dbl, "AD3"=w272:dbl, "AD4"=w271:dbl, "AD5"=w270:dbl)
            n144 = call <vilib>:"Read Coils.vi"("error in (no error)"=w259, "quantity"=u16 32 ("number of coils"), "starting address"=u16 0, "MB session in"=w260) -> ("error out"=w255:errorcluster, "Coils"=w244:bool[], "MB session out"=w256:refnum<class "MB_Master.lvclass">)  [unwired: 5 in]
            n145 = Bundle(w275, w274, w273, w272, w271, w270) -> (w276:cluster{dbl, dbl, dbl, dbl, dbl, dbl})  [unwired: 1 in]
            n146 = global write "采配水全局变量.vi" "输出状态"(w244) -> ()
            n147 = global write "采配水全局变量.vi" "转换值"(w276) -> ()
            n148 = call <vilib>:"Read Coils.vi"("error in (no error)"=w255, "quantity"=u16 16 ("number of coils"), "starting address"=u16 1000, "MB session in"=w256) -> ("error out"=w251:errorcluster, "Coils"=w245:bool[], "MB session out"=w252:refnum<class "MB_Master.lvclass">)  [unwired: 5 in]
            n149 = Index Array(array=w244, index #13=17 ("索引")) -> (element #1=w234:bool, element #2=w233:bool, element #3=w232:bool, element #4=w231:bool, element #5=w230:bool, element #6=w229:bool, element #7=w228:bool, element #8=w227:bool, element #9=w226:bool, element #10=w225:bool, element #11=w224:bool, element #12=w223:bool, element #13=w221:bool)  [unwired: 13 in, 1 out]
            n150 = local write "V13NO"(w234) -> ()
            n151 = local write "V13NC"(w233) -> ()
            n152 = local write "V14NO"(w232) -> ()
            n153 = local write "V14NC"(w231) -> ()
            n154 = local write "V3"(w230) -> ()
            n155 = local write "V4"(w229) -> ()
            n156 = local write "V5"(w228) -> ()
            n157 = local write "V2"(w227) -> ()
            n158 = local write "V6"(w226) -> ()
            n159 = local write "M1-1"(w225) -> ()
            n160 = local write "M1-2"(w224) -> ()
            n161 = local write "M2"(w223) -> ()
            n162 = local write "进样阀"(w221) -> ()
            n163 = global write "采配水全局变量.vi" "输入状态"(w245) -> ()
            n164 = call <vilib>:"Read Coils.vi"("error in (no error)"=w251, "quantity"=u16 16 ("number of coils"), "starting address"=u16 2500, "MB session in"=w252) -> ("error out"=w246:errorcluster, "Coils"=w248:bool[], "MB session out"=w247:refnum<class "MB_Master.lvclass">)  [unwired: 5 in]
            n165 = Index Array(array=w245, index #3=6 ("索引")) -> (element #1=→"X0":bool, element #2=→"X1":bool, element #3=→"X6":bool)  [unwired: 2 in]
            n166 = global write "采配水全局变量.vi" "报警簇"(w248) -> ()
          }
          frame "读参数" {
            n167 = call <vilib>:"Read Holding Registers.vi"("error in (no error)"=w299, "quantity"=u16 20 ("number of holding registers"), "starting address"=u16 100, "MB session in"=w300) -> ("error out"=w294:errorcluster, "Registers"=w296:u16[], "MB session out"=w295:refnum<class "MB_Master.lvclass">)  [unwired: 5 in]
            n168 = Array To Cluster(array=w296) -> (cluster=w283:T18)
            n169 = global write "采配水全局变量.vi" "参数设置"(w283) -> ()
            n170 = Unbundle(w283) -> ("Registers[0]"=→"R100":u16, "Registers[1]"=→"R101":u16, "Registers[2]"=→"R102":u16, "Registers[3]"=→"R103":u16, "Registers[4]"=→"R104":u16, "Registers[5]"=→"R105":u16, "Registers[6]"=→"R106":u16, "Registers[7]"=→"R107":u16, "Registers[8]"=→"R108":u16, "Registers[9]"=→"R109":u16, "Registers[10]"=w282:u16, "Registers[11]"=→"R111":u16, "Registers[12]"=→"R112":u16, "Registers[13]"=→"R113":u16, "Registers[16]"=w278:u16)  [unwired: 19 out]
            n171 = local write "潜水泵工作模式"(w282) -> ()
            n172 = local write "R116"(w278) -> ()
          }
          frame "多个写入" {
            n173 = Unbundle By Name(w306) -> ("数据"=w305:variant)
            n174 = Variant To Data(type=T13 {"starting address"=0, "holding register values"=[]}, Variant=w305) -> (data=w303:T13)  [unwired: 1 in, 1 out]
            n175 = Unbundle By Name(w303) -> ("starting address"=w302:u16, "holding register values"=w301:u16[])
            n176 = call <vilib>:"Write Multiple Registers.vi"("error in (no error)"=w309, "values"=w301, "starting address"=w302, "MB session in"=w310) -> ("error out"=w308:errorcluster, "MB session out"=w307:refnum<class "MB_Master.lvclass">)  [unwired: 6 in]
          }
          frame "单个写入" {
            n177 = Unbundle By Name(w316) -> ("数据"=w315:variant)
            n178 = Variant To Data(type=T14 {"starting address"=0, "holding register value"=0}, Variant=w315) -> (data=w313:T14)  [unwired: 1 in, 1 out]
            n179 = Unbundle By Name(w313) -> ("starting address"=w312:u16, "holding register value"=w311:u16)
            n180 = call <vilib>:"Write Single Register.vi"("error in (no error)"=w319, "value"=w311, "address"=w312, "MB session in"=w320) -> ("error out"=w318:errorcluster, "MB session out"=w317:refnum<class "MB_Master.lvclass">)  [unwired: 6 in]
          }
          frame "线圈写入" {
            n181 = Unbundle By Name(w326) -> ("数据"=w325:variant)
            n182 = Variant To Data(type=T15 {"starting address"=0, "coil values"=[]}, Variant=w325) -> (data=w323:T15)  [unwired: 1 in, 1 out]
            n183 = Unbundle By Name(w323) -> ("starting address"=w322:u16, "coil values"=w321:bool[])
            n184 = call <vilib>:"Write Multiple Coils.vi"("error in (no error)"=w329, "values"=w321, "starting address"=w322, "MB session in"=w330) -> ("error out"=w328:errorcluster, "MB session out"=w327:refnum<class "MB_Master.lvclass">)  [unwired: 6 in]
          }
          frame "shutdown" {
            n185 = call <vilib>:"Write Single Register.vi"("error in (no error)"=w334, "value"=u16 0, "address"=u16 4047, "MB session in"=w333) -> ("error out"=w335:errorcluster, "MB session out"=w338:refnum<class "MB_Master.lvclass">)  [unwired: 6 in]
            n186 = call-dynamic "Close Session.vi"("error in (no error)"=w335, "MB session in"=w338) -> ("error out"=w339:errorcluster)  [unwired: 9 in]
            n187 = call <vilib>:"Clear Errors.vi"("error in (no error)"=w339) -> ("error out"=w332:errorcluster)  [unwired: 5 in, 1 out]
            n188 = call "调用WinProladder.vi"("错误输入（无错误）"=w332) -> ("错误输出"=w331:errorcluster)  [unwired: 10 in]
          }
        }
      }
      frame Error {
        n189 = Unbundle By Name(w345) -> ("code"=w347:i32)
        n190 = case shown="-1073807343" w347 {
          tunnel: w346 -> [w349 w353]
          tunnel: w345 -> [w348 w355]
          tunnel: [w348 w354] -> w343
          tunnel: [w349 w353] -> w344
          tunnel: w341 -> [_ w352]
          frame Default {
          }
          frame -1073807343 {
            n191 = Flush Queue(queue=w352) -> (queue out=w351:refnum<queue>)  [unwired: 1 in, 2 out]
            n192 = call-dynamic "Close Session.vi"("error in (no error)"=w355, "MB session in"=w353) -> ("error out"=w354:errorcluster)  [unwired: 9 in]
            n193 = disable-structure shown="禁用" {
              disable-tunnel: w351 -> [w356 _]
              frame Disabled {
                n194 = Enqueue Element At Opposite End(queue=w356, element=cluster{"命令":string, "数据":variant} {"命令"="init", "数据"=variant} ("元素")) -> ()  [unwired: 2 in, 3 out]
              }
              frame Enabled {
              }
            }
            n195 = Wait (ms)(milliseconds to wait=u32 2000 ("等待时间（毫秒）")) -> ()  [unwired: 1 out]
          }
        }
        n196 = call <vilib>:"Clear Errors.vi"("error in (no error)"=w343) -> ("error out"=w342:errorcluster)  [unwired: 5 in, 1 out]
      }
    }
    n197 = Unbundle By Name(w191) -> ("status"=→"通讯故障":bool)
  }
  n198 = property on="多列列表框" class="MCListbox (严格)"("ItemNames"=string[][] [["待机"], ["初始化"], ["外部管路润洗"], ["内部管路润洗"], ["采样"], ["沉淀"], ["配水"], ["外部管路反冲洗"], ["内部管路反冲洗"], ["采样池储水"], ["结束"]] ("项名")) -> ()  [unwired: 2 in, 2 out]
  n199 = call-dynamic "Close Session.vi"("error in (no error)"=w5, "MB session in"=w4) -> ()  [unwired: 9 in, 1 out]
